vi "fpga_LP1 ControlUnit.vi"(0 "#Ch":fxp<+,5,5>=16.0, 1 "reset":bool, 2 "input valid":bool) -> (5 "ready for input":bool, 6 "procInputValid":bool, 7 "output valid":bool, 8 "opState":T1, 9 "coefRDAddr":fxp<+,6,6>)   [LabVIEW 2011, in "NI_EP_PMU_FPGA.lvlib"]
uses:
  <vilib>/addons/Electrical Power/PMU/NI_EP_PMU_FPGA.lvlib
  <vilib>/rvi/FXPMathLib/basic elements/FxpDiscreteDelay/XNode/nifxpmath_DiscreteDelay.xnode
  <vilib>/rvi/FXPMathLib/basic elements/FxpAddSub/XNode/nifxpmath_AddSub.xnode
  <vilib>/rvi/FXPMathLib/sim/FxpSim.dll
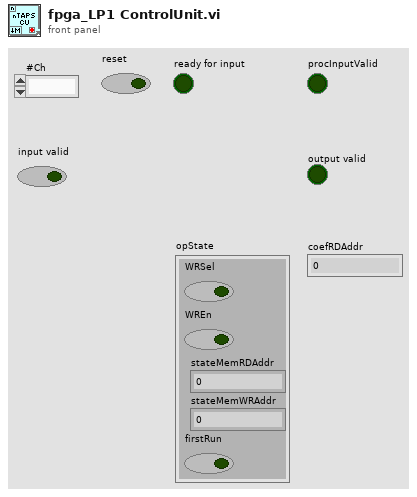
[diagram p1: front panel]
types:
  T1 = cluster{"WRSel":bool, "WREn":bool, "stateMemRDAddr":fxp<+,7,7>, "stateMemWRAddr":fxp<+,7,7>, "firstRun":bool}
  T2 = cluster{"idle":bool, "ready for input":bool, "macCnt":fxp<+,3,3>, "chCnt":fxp<+,5,5>, "phaseCnt":fxp<+,4,4>, "WRPageAddr":fxp<+,7,7>, "WRBaseAddr":fxp<+,7,7>, "first run?":bool}
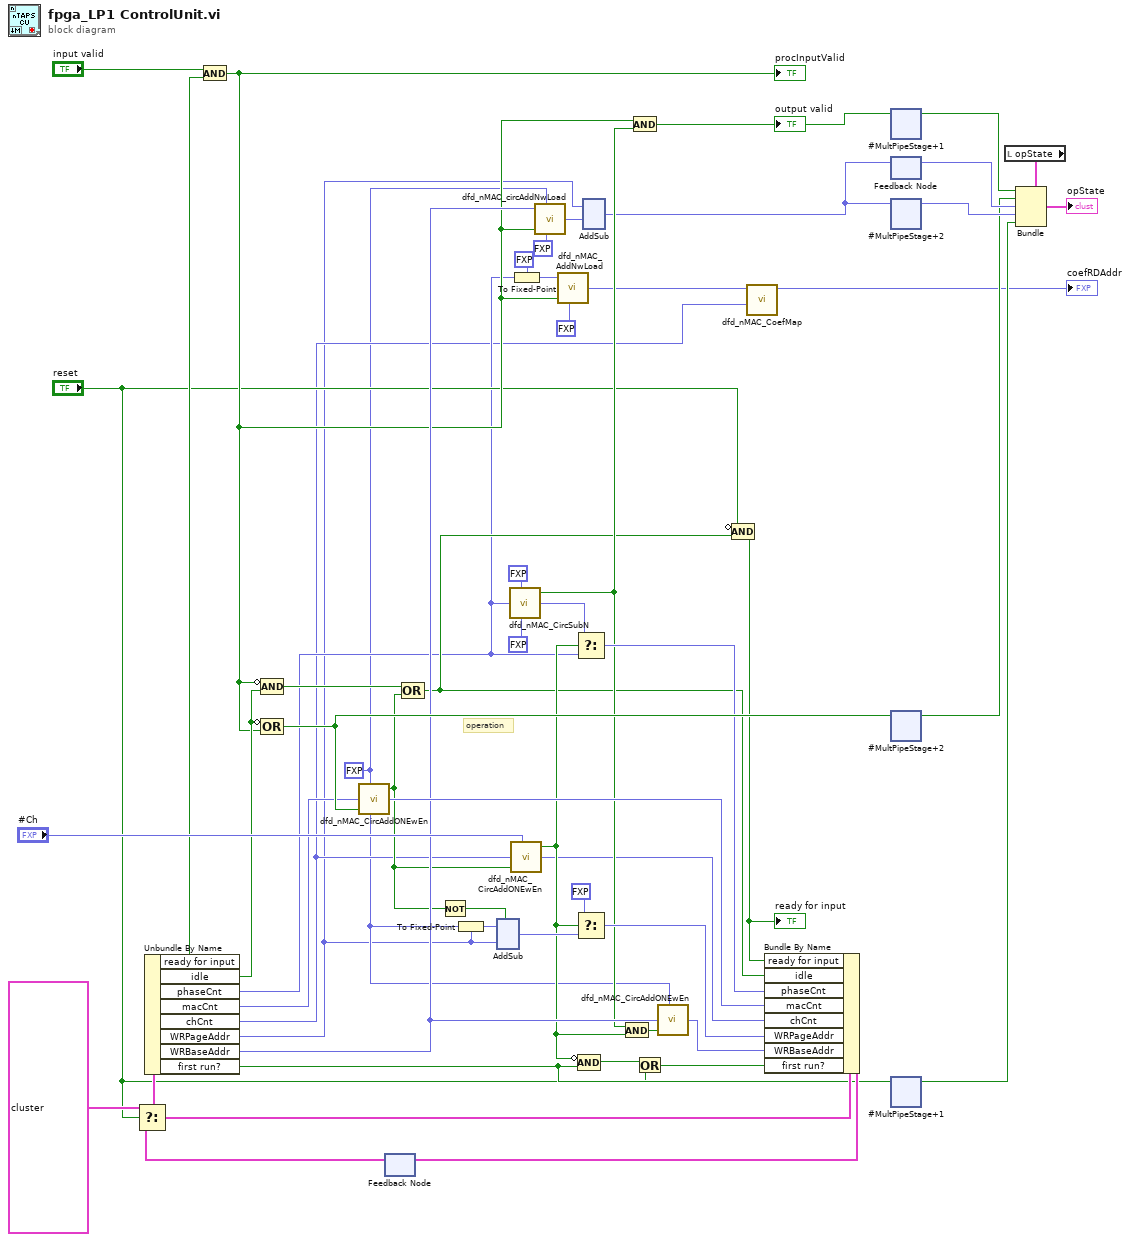
[diagram p0: block diagram]
diagram:
  w3 = fxp<+,3,3> 7.0 ("#TPPM")
  # "operation"
  n1 = feedback #1() -> (w39:T2)  [unwired: 1 out]
  n2 = Select(t=T2 {"idle"=TRUE, "ready for input"=FALSE, "macCnt"=0.0, "chCnt"=0.0, "phaseCnt"=0.0, "WRPageAddr"=0.0, "WRBaseAddr"=0.0, "first run?"=TRUE} ("CUInitialState"), s="reset", f=w39) -> (s? t:f=w41:T2)
  n3 = Unbundle By Name(w41) -> ("ready for input"=w23:bool, "idle"=w30:bool, "phaseCnt"=w10:fxp<+,4,4>, "macCnt"=w37:fxp<+,3,3>, "chCnt"=w4:fxp<+,5,5>, "WRPageAddr"=w1:fxp<+,7,7>, "WRBaseAddr"=w34:fxp<+,7,7>, "first run?"=w18:bool)
  n4 = And(x="input valid", y=w23) -> (x .and. y?=w22:bool)
  "procInputValid" <- w22
  n5 = Compound Arithmetic op=AND(invert w22, w30) -> (w47:bool)
  n6 = Compound Arithmetic op=OR(invert w30, w22) -> (w44:bool)
  n7 = call "dfd_nMAC_CircAddONEwEn.vi"("len"=w3, "idxIn"=w37, "Enable"=w44) -> ("wrap?"=w19:bool, "idxOut"=w36:fxp<+,3,3>)  [unwired: 5 in]
  n8 = Compound Arithmetic op=OR(w47, w19) -> (w20:bool)
  n9 = Not(x=w19) -> (.not. x?=w52:bool)
  n10 = To Fixed-Point ("ToCoef")(fixed-point type=w1, number=w3) -> (fixed-point=w2:fxp<+,7,7>)
  n11 = xnode ("AddSub")("x"=w2, "y"=w1, "use zero instead of x"=w52) -> ("s"=w50:fxp<+,7,7>)  [unwired: 1 out]
  n12 = call "dfd_nMAC_CircSubN.vi"("len"=fxp<+,4,4> 8.0 ("#M"), "idxIn"=w10, "step"=fxp<+,1,1> 1.0 ("#L")) -> ("wrap?"=w32:bool, "idxOut"=w31:fxp<+,4,4>)  [unwired: 5 in]
  n13 = call "dfd_nMAC_CircAddONEwEn.vi"("len"="#Ch", "idxIn"=w4, "Enable"=w19) -> ("wrap?"=w28:bool, "idxOut"=w21:fxp<+,5,5>)  [unwired: 5 in]
  n14 = To Fixed-Point ("ToCoef")(fixed-point type=fxp<+,6,6> 0.0 ("CoefAddr"), number=w10) -> (fixed-point=w12:fxp<+,6,6>)
  n15 = call "dfd_nMAC_circAddNwLoad.vi"("initIdx"=w34, "len"=w3, "load"=w22, "step"=fxp<+,1,1> 1.0) -> ("idxOut"=w14:fxp<+,7,7>)  [unwired: 5 in]
  n16 = call "dfd_nMAC_AddNwLoad.vi"("initIdx"=w12, "load"=w22, "step"=fxp<+,4,4> 8.0 ("#M")) -> ("idxOut"=w6:fxp<+,6,6>)  [unwired: 6 in]
  n17 = Select(t=w31, s=w28, f=w10) -> (s? t:f=w38:fxp<+,4,4>)
  n18 = Select(t=fxp<+,1,1> 0.0, s=w28, f=w50) -> (s? t:f=w35:fxp<+,7,7>)
  n19 = Compound Arithmetic op=AND(invert w28, w18) -> (w26:bool)
  n20 = xnode ("AddSub")("x"=w1, "y"=w14) -> ("s"=w13:fxp<+,7,7>)  [unwired: 1 out]
  n21 = And(x=w32, y=w28) -> (x .and. y?=w49:bool)
  n22 = And(x=w22, y=w32) -> (x .and. y?=w25:bool)
  "output valid" <- w25
  n23 = Or(x=w26, y="reset") -> (x .or. y?=w27:bool)
  n24 = call "dfd_nMAC_CircAddONEwEn.vi"("len"=w3, "idxIn"=w34, "Enable"=w49) -> ("idxOut"=w33:fxp<+,7,7>)  [unwired: 5 in, 1 out]
  n25 = Compound Arithmetic op=AND(invert "reset", w20) -> (w16:bool)
  "ready for input" <- w16
  n26 = call "dfd_nMAC_CoefMap.vi"("chCnt"=w4, "coefOffsetAddr"=w6) -> ("coefRDAddr"=→"coefRDAddr":fxp<+,6,6>)  [unwired: 9 in]
  n27 = Bundle By Name(cluster=w41, "ready for input"=w16, "idle"=w20, "phaseCnt"=w38, "macCnt"=w36, "chCnt"=w21, "WRPageAddr"=w35, "WRBaseAddr"=w33, "first run?"=w27) -> (w40:T2)
  n28 = feedback-in #1(w40) -> ()
  n29 = xnode ("#MultPipeStage+1")("D"=w25) -> ("Q"=w24:bool)
  n30 = feedback-in #2(w13) -> ()
  n31 = feedback #2() -> (w46:fxp<+,7,7>)  [unwired: 1 out]
  n32 = xnode ("#MultPipeStage+2")("D"=w13) -> ("Q"=w45:fxp<+,7,7>)
  n33 = xnode ("#MultPipeStage+2")("D"=w44) -> ("Q"=w43:bool)
  n34 = xnode ("#MultPipeStage+1")("D"=w18) -> ("Q"=w7:bool)
  n35 = local read "opState"() -> (w9:T1)
  n36 = Bundle(cluster=w9, "WRSel"=w24, "WREn"=w43, "stateMemRDAddr"=w46, "stateMemWRAddr"=w45, "firstRun"=w7) -> (→"opState":T1)
